vi "Data Message Decoding.vi"(8 "error in":errorcluster, 10 "Message Text":u8[](array[numeric]), 11 "SECS-II Class in":refnum<class "SECS-II Class.lvclass">) -> (0 "error out":errorcluster, 2 "Error?":bool, 3 "SECS-II Class out":refnum<class "SECS-II Class.lvclass">)   [LabVIEW 2020, in "SECS Communication.lvlib" / "SECS-II Class.lvclass"]
uses:
  SECS-II Class.lvclass
  Data Item Format.ctl
  Format Code.ctl
  Message Data.ctl
  SECS-II Class.lvclass/SECS-II Class.ctl
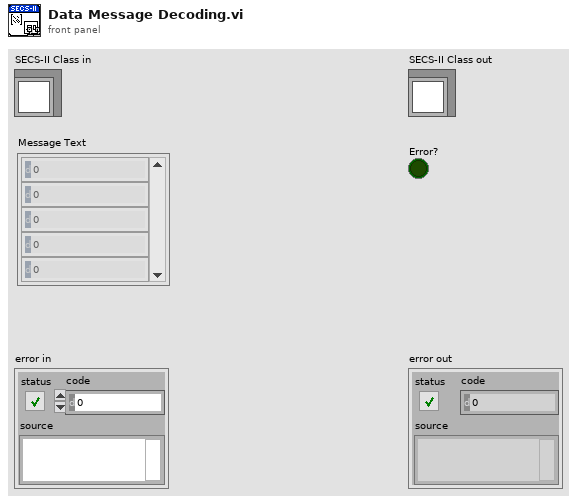
[diagram p1: front panel]
types:
  T1 = typedef "SECS Communication.lvlib/SECS-II Class.lvclass/Data Item Format.ctl" = enum16{"Data Type", "Value"}
  T2 = typedef "SECS Communication.lvlib/SECS-II Class.lvclass/Format Code.ctl" = enum16{"L", "A", "B", "Boolean", "J", "I1", "I2", "I4", "I8", "U1", "U2", "U4", "U8", "F4", "F8", "Char"}
  T3 = cluster{"Index":i32, "Data Item Format":T1, "Count":i32, "Error?":bool, "Data Length":u32, "Format Code":T2, "Data Index":i32, "Parent Index":i32[], "Correct":bool, "Over":bool}
  T4 = typedef "SECS Communication.lvlib/SECS-II Class.lvclass/Message Data.ctl" = cluster{"Index":i32, "Data Item Format":T1, "Format Code":T2, "Parent Index":i32, "Child Index":i32[], "Data":variant}
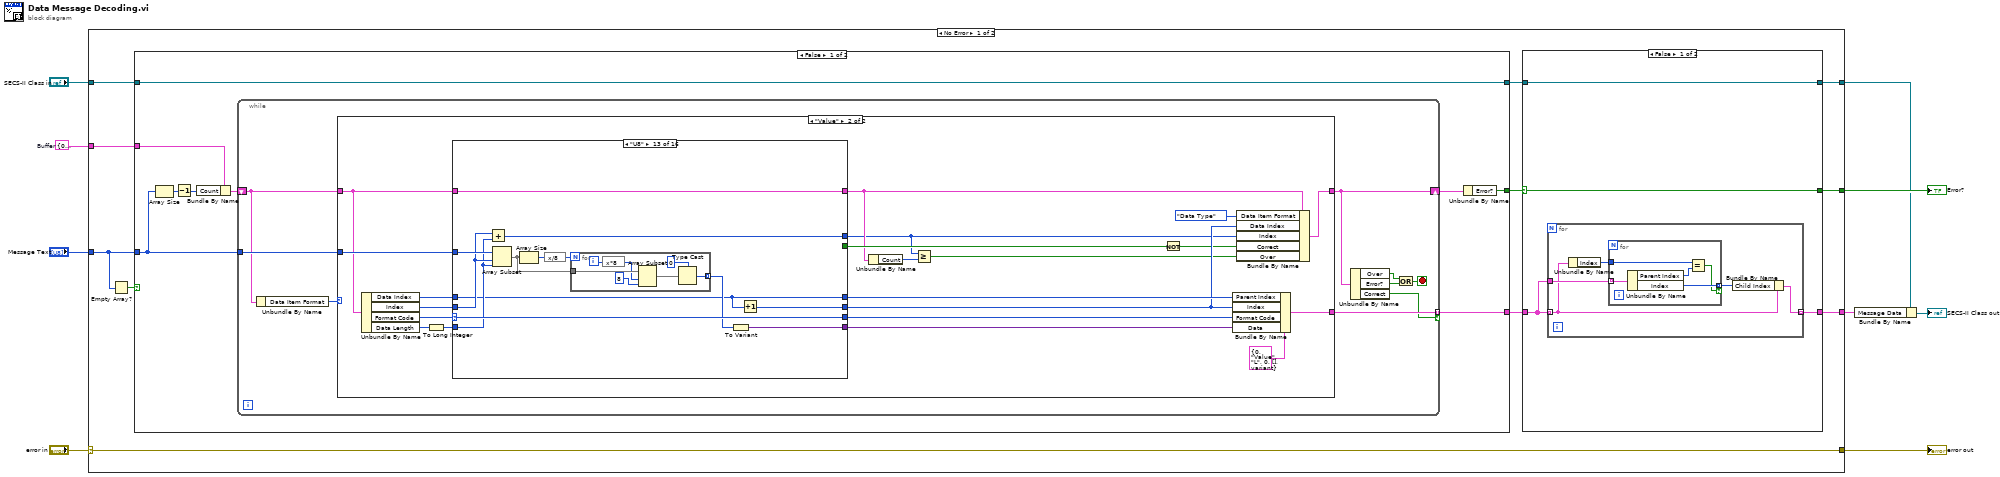
[diagram p0: block diagram]
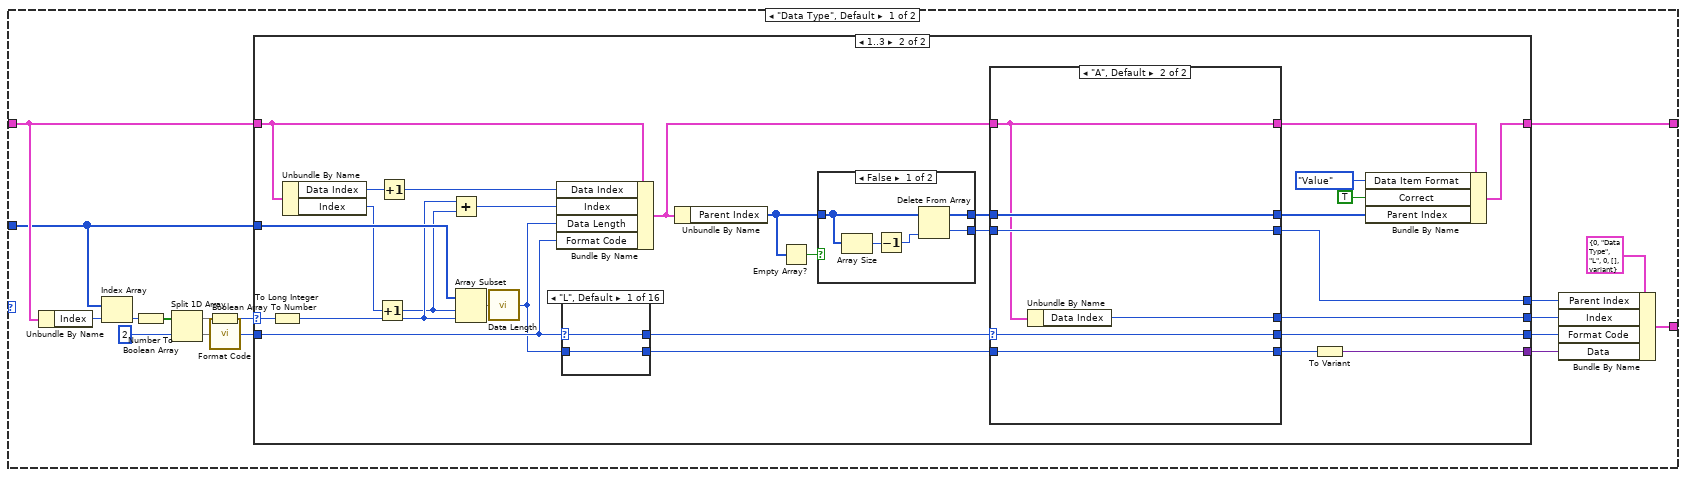
[diagram p3: hidden frame]
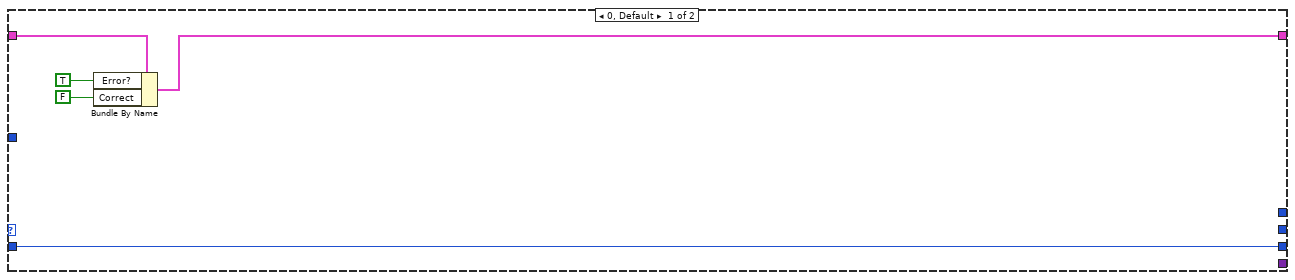
[diagram p4: hidden frame]
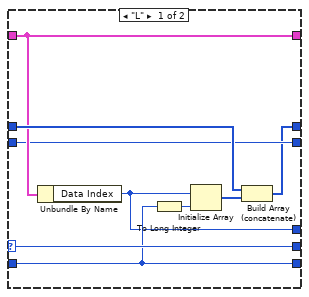
[diagram p5: hidden frame]
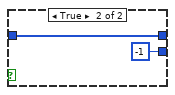
[diagram p6: hidden frame]
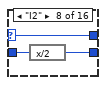
[diagram p13: hidden frame]
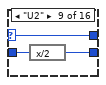
[diagram p14: hidden frame]
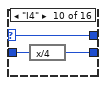
[diagram p15: hidden frame]
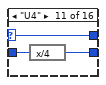
[diagram p16: hidden frame]
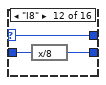
[diagram p17: hidden frame]
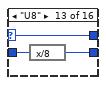
[diagram p18: hidden frame]
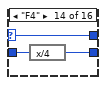
[diagram p19: hidden frame]
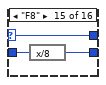
[diagram p20: hidden frame]
diagram:
  w6 = T3 {"Index"=0, "Data Item Format"=enum."Data Type", "Count"=0, "Error?"=FALSE, "Data Length"=0, "Format Code"=enum."L", "Data Index"=-1, "Parent Index"=[], "Correct"=FALSE, "Over"=FALSE}  # Buffer
  n1 = case shown="No Error" "error in" {
    selector: "error in" -> [w19 w439]
    tunnel: [w19 w439] -> w7
    tunnel: "Message Text" -> [w18 _]
    tunnel: [w14 _] -> w2
    tunnel: w6 -> [w17 _]
    tunnel: [w13 TRUE] -> w5
    tunnel: "SECS-II Class in" -> [w12 w437]
    tunnel: [w10 w437] -> w3
    frame No Error {
      n2 = Empty Array?(array=w18) -> (empty?=w20:bool)
      n3 = case shown="False" w20 {
        tunnel: w18 -> [w45 _]
        tunnel: [w44 _] -> w15
        tunnel: w17 -> [w43 _]
        tunnel: [w41 _] -> w16
        tunnel: w12 -> [w40 w436]
        tunnel: [w40 w436] -> w11
        frame False {
          n4 = Array Size(array=w45) -> (size(s)=w38:i32)
          n5 = Decrement(x=w38) -> (x-1=w39:i32)
          n6 = Bundle By Name(cluster=w43, "Count"=w39) -> (w46:T3)
          n7 = while {
            tunnel: w45 -> [w54]
            shift-right: [w51] -> w42
            shift-left: w46 -> [w53]
            tunnel: [w52] -> w44 mode=indexing if=w49
            stop <- w48 stop-if-true
            n8 = Unbundle By Name(w53) -> ("Data Item Format"=w55:T1)
            n9 = case shown="\"Value\"" w55 {
              tunnel: w54 -> [w60 w189]
              tunnel: w53 -> [w65 w177]
              tunnel: [w63 w187] -> w51
              tunnel: [w61 w183] -> w52
              frame "Data Type", Default {
                n10 = Unbundle By Name(w65) -> ("Index"=w72:i32)
                n11 = Index Array(array=w60, index=w72) -> (element=w71:u8)
                n12 = Number To Boolean Array(number=w71) -> (Boolean array=w70:bool[])
                n13 = Split 1D Array(array=w70, index=2) -> (first subarray=w68:bool[], second subarray=w67:bool[])
                n14 = Boolean Array To Number(Boolean array=w68) -> (number=w66:u32)
                n15 = call "Format Code.vi"("Formay Code"=w67) -> ("Format Code"=w64:T2)
                n16 = case shown="1..3" w66 {
                  selector: w66 -> [_ w106]
                  tunnel: w65 -> [w77 w96]
                  tunnel: [w76 w87] -> w63
                  tunnel: w64 -> [w75 w101]
                  tunnel: [w75 w90] -> w62
                  tunnel: w60 -> [_ w105]
                  tunnel: [_ w84] -> w58
                  tunnel: [_ w83] -> w57
                  tunnel: [_ w80] -> w56
                  frame 0, Default {
                    n17 = Bundle By Name(cluster=w77, "Error?"=TRUE, "Correct"=FALSE) -> (w76:T3)
                  }
                  frame 1..3 {
                    n18 = To Long Integer(number=w106) -> (32bit integer=w102:i32)
                    n19 = Unbundle By Name(w96) -> ("Data Index"=w99:i32, "Index"=w79:i32)
                    n20 = Increment(x=w79) -> (x+1=w78:i32)
                    n21 = Increment(x=w99) -> (x+1=w98:i32)
                    n22 = Add(x=w102, y=w78) -> (x+y=w103:i32)
                    n23 = Array Subset(array=w105, index=w78, length=w102) -> (w104:u8[])
                    n24 = call "Data Length.vi"("Data Length U8 []"=w104) -> ("Data Length"=w100:u32)
                    n25 = Bundle By Name(cluster=w96, "Data Index"=w98, "Index"=w103, "Data Length"=w100, "Format Code"=w101) -> (w82:T3)
                    n26 = case shown="\"L\", Default" w101 {
                      selector: w101 -> [w130 w132 w134 w136 w138 w140 w142 w145 w148 w151 w154 w157 w160 w163 w166 w169]
                      tunnel: [w130 w132 w134 w136 w138 w140 w142 w145 w148 w151 w154 w157 w160 w163 w166 w169] -> w94
                      tunnel: w100 -> [w129 w131 w133 w135 w137 w139 w141 w144 w147 w150 w153 w156 w159 w162 w165 w168]
                      tunnel: [w129 w131 w133 w135 w137 w139 w141 w143 w146 w149 w152 w155 w158 w161 w164 w167] -> w93
                      frame "L", Default {
                      }
                      frame "A" {
                      }
                      frame "B" {
                      }
                      frame "Boolean" {
                      }
                      frame "J" {
                      }
                      frame "I1" {
                      }
                      frame "U1" {
                      }
                      frame "I2" {
                        n27 = expression code="x/2"(w144) -> (w143:u32)
                      }
                      frame "U2" {
                        n28 = expression code="x/2"(w147) -> (w146:u32)
                      }
                      frame "I4" {
                        n29 = expression code="x/4"(w150) -> (w149:u32)
                      }
                      frame "U4" {
                        n30 = expression code="x/4"(w153) -> (w152:u32)
                      }
                      frame "I8" {
                        n31 = expression code="x/8"(w156) -> (w155:u32)
                      }
                      frame "U8" {
                        n32 = expression code="x/8"(w159) -> (w158:u32)
                      }
                      frame "F4" {
                        n33 = expression code="x/4"(w162) -> (w161:u32)
                      }
                      frame "F8" {
                        n34 = expression code="x/8"(w165) -> (w164:u32)
                      }
                      frame "Char" {
                        n35 = expression code="x/2"(w168) -> (w167:u32)
                      }
                    }
                    n36 = Unbundle By Name(w82) -> ("Parent Index"=w95:i32[])
                    n37 = Empty Array?(array=w95) -> (empty?=w97:bool)
                    n38 = case shown="False" w97 {
                      tunnel: w95 -> [w126 w128]
                      tunnel: [w124 w128] -> w92
                      tunnel: [w123 -1 ("Numeric")] -> w91
                      frame False {
                        n39 = Array Size(array=w126) -> (size(s)=w125:i32)
                        n40 = Decrement(x=w125) -> (x-1=w122:i32)
                        n41 = Delete From Array(array=w126, index=w122) -> (deleted portion=w123:i32, array with subset deleted=w124:i32[])  [unwired: 1 in]
                      }
                      frame True {
                      }
                    }
                    n42 = case shown="\"A\", Default" w94 {
                      selector: w94 -> [w115 w120]
                      tunnel: w93 -> [w114 w121]
                      tunnel: w92 -> [w112 w119]
                      tunnel: w91 -> [w109 w118]
                      tunnel: w82 -> [w110 w117]
                      tunnel: [w115 w120] -> w90
                      tunnel: [w114 w121] -> w81
                      tunnel: [w110 w117] -> w89
                      tunnel: [w108 w119] -> w88
                      tunnel: [w109 w118] -> w83
                      tunnel: [w107 w116] -> w84
                      frame "L" {
                        n43 = Unbundle By Name(w110) -> ("Data Index"=w107:i32)
                        n44 = To Long Integer(number=w114) -> (32bit integer=w113:i32)
                        n45 = Initialize Array(w107, w113) -> (w111:i32[])
                        n46 = Build Array (concatenate)(w112, w111) -> (w108:i32[])
                      }
                      frame "A", Default {
                        n47 = Unbundle By Name(w117) -> ("Data Index"=w116:i32)
                      }
                    }
                    n48 = To Variant(anything=w81) -> (Variant=w80:variant)
                    n49 = Bundle By Name(cluster=w89, "Data Item Format"=Data_Item_Format."Value", "Correct"=TRUE, "Parent Index"=w88) -> (w87:T3)
                  }
                }
                n50 = Bundle By Name(cluster=T4 {"Index"=0, "Data Item Format"=enum."Data Type", "Format Code"=enum."L", "Parent Index"=0, "Child Index"=[], "Data"=variant} ("Message Data"), "Parent Index"=w57, "Index"=w58, "Format Code"=w62, "Data"=w56) -> (w61:T4)
              }
              frame "Value" {
                n51 = Unbundle By Name(w177) -> ("Data Index"=w179:i32, "Index"=w182:i32, "Format Code"=w190:T2, "Data Length"=w186:u32)
                n52 = To Long Integer(number=w186) -> (32bit integer=w185:i32)
                n53 = case shown="\"U8\"" w190 {
                  selector: w190 -> [w196 w208 w219 w233 w243 w254 w264 w277 w297 w317 w337 w357 w377 w397 w417 w435]
                  tunnel: w189 -> [_ w206 w217 w231 w241 w252 w262 w275 w295 w315 w335 w355 w375 w395 w415 w433]
                  tunnel: w177 -> [w197 w207 w218 w232 w242 w253 w263 w276 w296 w316 w336 w356 w376 w396 w416 w434]
                  tunnel: [w197 w207 w218 w232 w242 w253 w263 w276 w296 w316 w336 w356 w376 w396 w416 w434] -> w172
                  tunnel: w185 -> [w193 w203 w215 w229 w239 w250 w260 w273 w293 w313 w333 w353 w373 w393 w413 w431]
                  tunnel: [w196 w208 w219 w233 w243 w254 w264 w277 w297 w317 w337 w357 w377 w397 w417 w435] -> w184
                  tunnel: w182 -> [w195 w204 w216 w230 w240 w251 w261 w274 w294 w314 w334 w354 w374 w394 w414 w432]
                  tunnel: [w194 w201 w214 w228 w238 w249 w259 w272 w292 w312 w332 w352 w372 w392 w412 w428] -> w181
                  tunnel: w179 -> [w192 w199 w211 w225 w235 w245 w256 w266 w286 w306 w326 w346 w366 w386 w406 w426]
                  tunnel: [w192 w200 w209 w223 w234 w244 w255 w265 w285 w305 w325 w345 w365 w385 w405 w425] -> w176
                  tunnel: [w192 w199 w211 w225 w235 w245 w256 w266 w286 w306 w326 w346 w366 w386 w406 w426] -> w178
                  tunnel: [w195 w198 w210 w224 w236 w246 w257 w267 w287 w307 w327 w347 w367 w387 w407 w427] -> w171
                  tunnel: [TRUE _ _ _ _ _ _ _ _ _ _ _ _ _ _ _] -> w175
                  frame "L" {
                    n54 = To Variant(anything=w193) -> (Variant=w194:variant)
                  }
                  frame "A", Default {
                    n55 = Add(x=w204, y=w203) -> (x+y=w198:i32)
                    n56 = Array Subset(array=w206, index=w204, length=w203) -> (w205:u8[])
                    n57 = Byte Array To String(unsigned byte array=w205) -> (string=w202:string)
                    n58 = To Variant(anything=w202) -> (Variant=w201:variant)
                    n59 = Increment(x=w199) -> (x+1=w200:i32)
                  }
                  frame "B" {
                    n60 = Add(x=w216, y=w215) -> (x+y=w210:i32)
                    n61 = Array Subset(array=w217, index=w216, length=w215) -> (w213:u8[])
                    n62 = for {
                      tunnel: w213 -> [w222] mode=indexing
                      tunnel: [w220] -> w212 mode=indexing
                      n63 = Number To Boolean Array(number=w222) -> (Boolean array=w221:bool[])
                      n64 = Bundle("Boolean array"=w221) -> (w220:cluster{"Boolean array":bool[]})  [unwired: 1 in]
                    }
                    n65 = To Variant(anything=w212) -> (Variant=w214:variant)
                    n66 = Increment(x=w211) -> (x+1=w209:i32)
                  }
                  frame "Boolean" {
                    n67 = Add(x=w230, y=w229) -> (x+y=w224:i32)
                    n68 = Array Subset(array=w231, index=w230, length=w229) -> (w227:u8[])
                    n69 = Not Equal To 0?(x=w227) -> (x != 0?=w226:bool[])
                    n70 = To Variant(anything=w226) -> (Variant=w228:variant)
                    n71 = Increment(x=w225) -> (x+1=w223:i32)
                  }
                  frame "J" {
                    n72 = Array Subset(array=w241, index=w240, length=w239) -> (w237:u8[])
                    n73 = Add(x=w240, y=w239) -> (x+y=w236:i32)
                    n74 = To Variant(anything=w237) -> (Variant=w238:variant)
                    n75 = Increment(x=w235) -> (x+1=w234:i32)
                  }
                  frame "I1" {
                    n76 = Add(x=w251, y=w250) -> (x+y=w246:i32)
                    n77 = Array Subset(array=w252, index=w251, length=w250) -> (w248:u8[])
                    n78 = To Byte Integer(number=w248) -> (8bit integer=w247:i8[])
                    n79 = To Variant(anything=w247) -> (Variant=w249:variant)
                    n80 = Increment(x=w245) -> (x+1=w244:i32)
                  }
                  frame "U1" {
                    n81 = Add(x=w261, y=w260) -> (x+y=w257:i32)
                    n82 = Array Subset(array=w262, index=w261, length=w260) -> (w258:u8[])
                    n83 = To Variant(anything=w258) -> (Variant=w259:variant)
                    n84 = Increment(x=w256) -> (x+1=w255:i32)
                  }
                  frame "I2" {
                    n85 = Add(x=w274, y=w273) -> (x+y=w267:i32)
                    n86 = Array Subset(array=w275, index=w274, length=w273) -> (w269:u8[])
                    n87 = Array Size(array=w269) -> (size(s)=w271:i32)
                    n88 = expression code="x/2"(w271) -> (w270:i32)
                    n89 = for {
                      N: w270 -> [_]
                      tunnel: w269 -> [w284]
                      tunnel: [w278] -> w268 mode=indexing
                      i -> [w283]
                      n90 = expression code="x*2"(w283) -> (w282:i32)
                      n91 = Index Array(array=w284, index #1=w282) -> (element #1=w280:u8, element #2=w281:u8)  [unwired: 1 in]
                      n92 = Join Numbers(hi=w280, lo=w281) -> ((hi.lo)=w279:u16)
                      n93 = To Word Integer(number=w279) -> (16bit integer=w278:i16)
                    }
                    n94 = To Variant(anything=w268) -> (Variant=w272:variant)
                    n95 = Increment(x=w266) -> (x+1=w265:i32)
                  }
                  frame "U2" {
                    n96 = Add(x=w294, y=w293) -> (x+y=w287:i32)
                    n97 = Array Subset(array=w295, index=w294, length=w293) -> (w289:u8[])
                    n98 = Array Size(array=w289) -> (size(s)=w291:i32)
                    n99 = expression code="x/2"(w291) -> (w290:i32)
                    n100 = for {
                      N: w290 -> [_]
                      tunnel: w289 -> [w304]
                      tunnel: [w298] -> w288 mode=indexing
                      i -> [w303]
                      n101 = expression code="x*2"(w303) -> (w302:i32)
                      n102 = Index Array(array=w304, index #1=w302) -> (element #1=w300:u8, element #2=w301:u8)  [unwired: 1 in]
                      n103 = Join Numbers(hi=w300, lo=w301) -> ((hi.lo)=w299:u16)
                      n104 = To Unsigned Word Integer(number=w299) -> (unsigned 16bit integer=w298:u16)
                    }
                    n105 = To Variant(anything=w288) -> (Variant=w292:variant)
                    n106 = Increment(x=w286) -> (x+1=w285:i32)
                  }
                  frame "I4" {
                    n107 = Add(x=w314, y=w313) -> (x+y=w307:i32)
                    n108 = Array Subset(array=w315, index=w314, length=w313) -> (w309:u8[])
                    n109 = Array Size(array=w309) -> (size(s)=w311:i32)
                    n110 = expression code="x/4"(w311) -> (w310:i32)
                    n111 = for {
                      N: w310 -> [_]
                      tunnel: w309 -> [w324]
                      tunnel: [w318] -> w308 mode=indexing
                      i -> [w323]
                      n112 = expression code="x*4"(w323) -> (w322:i32)
                      n113 = Array Subset(array=w324, index=w322, length=4) -> (w320:u8[])
                      n114 = Type Cast(type=0, x=w320) -> (*(type *) &x=w318:i32)
                    }
                    n115 = To Variant(anything=w308) -> (Variant=w312:variant)
                    n116 = Increment(x=w306) -> (x+1=w305:i32)
                  }
                  frame "U4" {
                    n117 = Add(x=w334, y=w333) -> (x+y=w327:i32)
                    n118 = Array Subset(array=w335, index=w334, length=w333) -> (w329:u8[])
                    n119 = Array Size(array=w329) -> (size(s)=w331:i32)
                    n120 = expression code="x/4"(w331) -> (w330:i32)
                    n121 = for {
                      N: w330 -> [_]
                      tunnel: w329 -> [w344]
                      tunnel: [w338] -> w328 mode=indexing
                      i -> [w343]
                      n122 = expression code="x*4"(w343) -> (w342:i32)
                      n123 = Array Subset(array=w344, index=w342, length=4) -> (w340:u8[])
                      n124 = Type Cast(type=u32 0, x=w340) -> (*(type *) &x=w338:u32)
                    }
                    n125 = To Variant(anything=w328) -> (Variant=w332:variant)
                    n126 = Increment(x=w326) -> (x+1=w325:i32)
                  }
                  frame "I8" {
                    n127 = Add(x=w354, y=w353) -> (x+y=w347:i32)
                    n128 = Array Subset(array=w355, index=w354, length=w353) -> (w349:u8[])
                    n129 = Array Size(array=w349) -> (size(s)=w351:i32)
                    n130 = expression code="x/8"(w351) -> (w350:i32)
                    n131 = for {
                      N: w350 -> [_]
                      tunnel: w349 -> [w364]
                      tunnel: [w358] -> w348 mode=indexing
                      i -> [w363]
                      n132 = expression code="x*8"(w363) -> (w362:i32)
                      n133 = Array Subset(array=w364, index=w362, length=8) -> (w360:u8[])
                      n134 = Type Cast(type=i64 0, x=w360) -> (*(type *) &x=w358:i64)
                    }
                    n135 = To Variant(anything=w348) -> (Variant=w352:variant)
                    n136 = Increment(x=w346) -> (x+1=w345:i32)
                  }
                  frame "U8" {
                    n137 = Add(x=w374, y=w373) -> (x+y=w367:i32)
                    n138 = Array Subset(array=w375, index=w374, length=w373) -> (w369:u8[])
                    n139 = Array Size(array=w369) -> (size(s)=w371:i32)
                    n140 = expression code="x/8"(w371) -> (w370:i32)
                    n141 = for {
                      N: w370 -> [_]
                      tunnel: w369 -> [w384]
                      tunnel: [w378] -> w368 mode=indexing
                      i -> [w383]
                      n142 = expression code="x*8"(w383) -> (w382:i32)
                      n143 = Array Subset(array=w384, index=w382, length=8) -> (w380:u8[])
                      n144 = Type Cast(type=u64 0, x=w380) -> (*(type *) &x=w378:u64)
                    }
                    n145 = To Variant(anything=w368) -> (Variant=w372:variant)
                    n146 = Increment(x=w366) -> (x+1=w365:i32)
                  }
                  frame "F4" {
                    n147 = Add(x=w394, y=w393) -> (x+y=w387:i32)
                    n148 = Array Subset(array=w395, index=w394, length=w393) -> (w389:u8[])
                    n149 = Array Size(array=w389) -> (size(s)=w391:i32)
                    n150 = expression code="x/4"(w391) -> (w390:i32)
                    n151 = for {
                      N: w390 -> [_]
                      tunnel: w389 -> [w404]
                      tunnel: [w398] -> w388 mode=indexing
                      i -> [w403]
                      n152 = expression code="x*4"(w403) -> (w402:i32)
                      n153 = Array Subset(array=w404, index=w402, length=4) -> (w400:u8[])
                      n154 = Type Cast(type=sgl 0.0, x=w400) -> (*(type *) &x=w398:sgl)
                    }
                    n155 = To Variant(anything=w388) -> (Variant=w392:variant)
                    n156 = Increment(x=w386) -> (x+1=w385:i32)
                  }
                  frame "F8" {
                    n157 = Add(x=w414, y=w413) -> (x+y=w407:i32)
                    n158 = Array Subset(array=w415, index=w414, length=w413) -> (w409:u8[])
                    n159 = Array Size(array=w409) -> (size(s)=w411:i32)
                    n160 = expression code="x/8"(w411) -> (w410:i32)
                    n161 = for {
                      N: w410 -> [_]
                      tunnel: w409 -> [w424]
                      tunnel: [w418] -> w408 mode=indexing
                      i -> [w423]
                      n162 = expression code="x*8"(w423) -> (w422:i32)
                      n163 = Array Subset(array=w424, index=w422, length=8) -> (w420:u8[])
                      n164 = Type Cast(type=0.0, x=w420) -> (*(type *) &x=w418:dbl)
                    }
                    n165 = To Variant(anything=w408) -> (Variant=w412:variant)
                    n166 = Increment(x=w406) -> (x+1=w405:i32)
                  }
                  frame "Char" {
                    n167 = Add(x=w432, y=w431) -> (x+y=w427:i32)
                    n168 = Array Subset(array=w433, index=w432, length=w431) -> (w430:u8[])
                    n169 = Byte Array To String(unsigned byte array=w430) -> (string=w429:string)
                    n170 = To Variant(anything=w429) -> (Variant=w428:variant)
                    n171 = Increment(x=w426) -> (x+1=w425:i32)
                  }
                }
                n172 = Unbundle By Name(w172) -> ("Count"=w173:i32)
                n173 = Greater Or Equal?(x=w171, y=w173) -> (x >= y?=w170:bool)
                n174 = Not(x=w175) -> (.not. x?=w174:bool)
                n175 = Bundle By Name(cluster=T4 {"Index"=0, "Data Item Format"=enum."Value", "Format Code"=enum."L", "Parent Index"=0, "Child Index"=[], "Data"=variant} ("Message Data"), "Parent Index"=w178, "Index"=w176, "Format Code"=w184, "Data"=w181) -> (w183:T4)
                n176 = Bundle By Name(cluster=w172, "Data Item Format"=Data_Item_Format."Data Type", "Data Index"=w176, "Index"=w171, "Correct"=w174, "Over"=w170) -> (w187:T3)
              }
            }
            n177 = Unbundle By Name(w51) -> ("Over"=w47:bool, "Error?"=w50:bool, "Correct"=w49:bool)
            n178 = Or(x=w47, y=w50) -> (x .or. y?=w48:bool)
          }
          n179 = Unbundle By Name(w42) -> ("Error?"=w41:bool)
        }
        frame True {
        }
      }
      n180 = case shown="False" w16 {
        selector: w16 -> [w23 w37]
        tunnel: w15 -> [w21 w36]
        tunnel: [w24 w36] -> w14
        tunnel: [w23 w37] -> w13
        tunnel: w11 -> [w22 w35]
        tunnel: [w22 w35] -> w10
        frame False {
          n181 = for {
            tunnel: w21 -> [w27] mode=indexing
            tunnel: w21 -> [w29]
            tunnel: [w25] -> w24 mode=indexing
            n182 = Unbundle By Name(w27) -> ("Index"=w28:i32)
            n183 = for {
              tunnel: w29 -> [w34] mode=indexing
              tunnel: w28 -> [w33]
              tunnel: [w31] -> w26 mode=indexing if=w30
              n184 = Unbundle By Name(w34) -> ("Parent Index"=w32:i32, "Index"=w31:i32)
              n185 = Equal?(x=w33, y=w32) -> (x = y?=w30:bool)
            }
            n186 = Bundle By Name(cluster=w27, "Child Index"=w26) -> (w25:T4)
          }
        }
        frame True {
        }
      }
    }
    frame Error {
    }
  }
  "error out" <- w7
  "Error?" <- w5
  n187 = Bundle By Name(cluster=w3, "Message Data"=w2) -> (→"SECS-II Class out":refnum<class "SECS-II Class.lvclass">)
